vi "Test Semaphore 2.vi"() -> ()   [LabVIEW 2011]
panel:
  out "Iterations":u32
  in  "milliseconds to Hold":u32=500
  in  "milliseconds to wait":u32=500
  out "Wait Time":u32
  out "Hold Time":u32
  out "millisecond timer value 1":u32
  out "Prior Count":i32
  out "millisecond timer value 2":u32
  out "Locked 1":bool
  out "Numeric":i32
  out "Timed Out? 1":bool
  out "error out rel 2":errorcluster
  out "error out acq 2":errorcluster
  in  "Acq":bool
  in  "Release":bool
  in  "stop":bool
  out "Handle":u16
  out "error out create":errorcluster
  in  "Name":string="LabVIEW_System_Semaphore"
  out "error out destroy 1":errorcluster
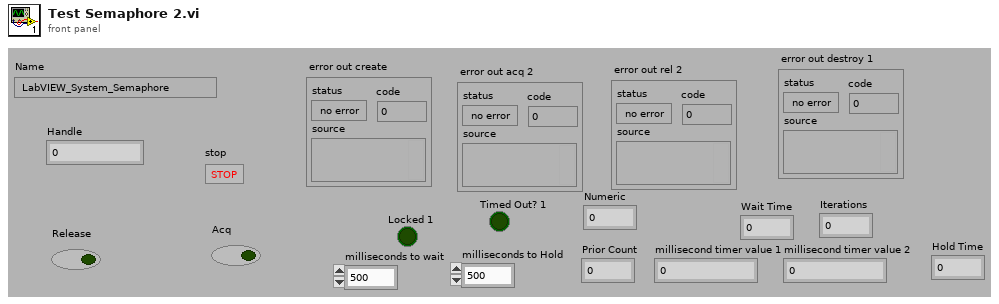
[diagram p1: front panel]
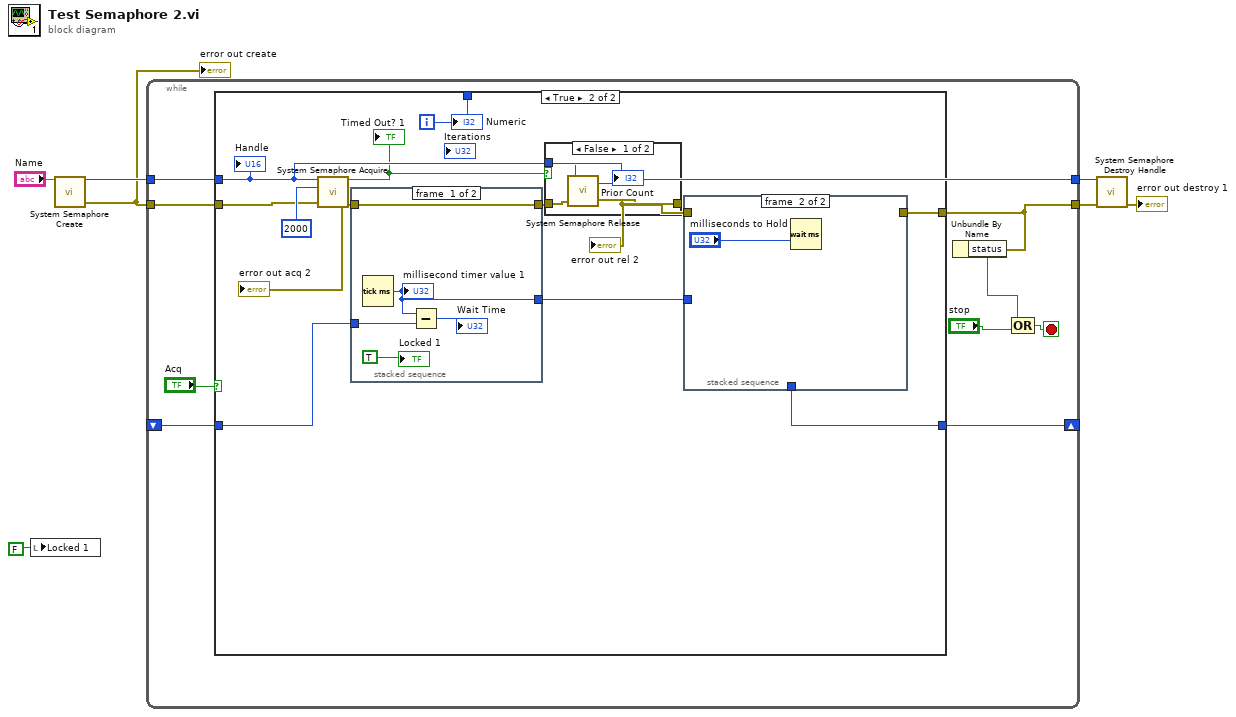
[diagram p0: block diagram]
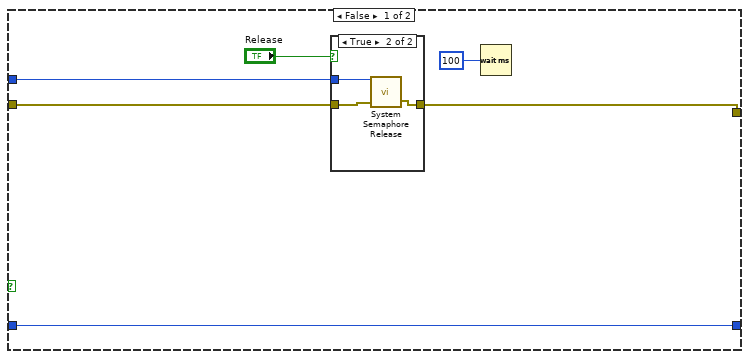
[diagram p2: hidden frame]
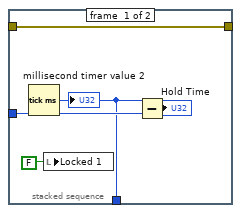
[diagram p5: hidden frame]
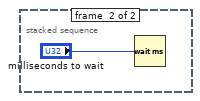
[diagram p6: hidden frame]
diagram:
  n1 = local write "Locked 1"(FALSE) -> ()
  n2 = call "System Semaphore Create.vi"("Name"="Name") -> ("error out"=w2:errorcluster, "Handle"=w7:u16)  [unwired: 4 in]
  "error out create" <- w2
  n3 = while {
    tunnel: w2 -> [w10]
    tunnel: w7 -> [w13]
    tunnel: [w13] -> w6
    tunnel: [w12] -> w5
    shift-right: [w9] -> _
    shift-left: _ -> [w8]
    i -> [w14]
    stop <- w16 stop-if-true
    n4 = case shown="True" "Acq" {
      tunnel: w14 -> [_ w39]
      tunnel: w13 -> [w19 w33]
      tunnel: [w20 w37] -> w12
      tunnel: w10 -> [w21 w32]
      tunnel: [w22 w30] -> w9
      tunnel: w8 -> [w22 w29]
      frame False {
        n5 = case shown="True" "Release" {
          tunnel: w21 -> [w24 w27]
          tunnel: [w24 w26] -> w20
          tunnel: w19 -> [_ w25]
          frame False {
          }
          frame True {
            n6 = call "System Semaphore Release.vi"("error in (no error)"=w27, "SemaphoreHandle"=w25) -> ("error out"=w26:errorcluster)  [unwired: 1 in, 1 out]
          }
        }
        n7 = Wait (ms)(milliseconds to wait=u32 100) -> ()  [unwired: 1 out]
      }
      frame True {
        n8 = call "System Semaphore Acquire.vi"("error in (no error)"=w32, "Timeout (ms)"=u16 2000, "SemaphoreHandle"=w33) -> ("error out"=w36:errorcluster, "Timed Out?"=w28:bool)
        "Timed Out? 1" <- w28
        "error out acq 2" <- w36
        n9 = stacked-sequence {
          tunnel: w36 -> [w55 _]
          tunnel: [w55 _] -> w35
          tunnel: [w52 _] -> w31
          tunnel: w29 -> [w51 _]
          frame #0 {
            n10 = Tick Count (ms)() -> (millisecond timer value=w52:u32)
            "millisecond timer value 1" <- w52
            n11 = Subtract(x=w52, y=w51) -> (x-y=→"Wait Time":u32)
            "Locked 1" <- TRUE
          }
          frame #1 {
            n12 = Wait (ms)(milliseconds to wait="milliseconds to wait") -> ()  [unwired: 1 out]
          }
        }
        n13 = case shown="False" w28 {
          tunnel: w35 -> [w43 w44]
          tunnel: w33 -> [w42 _]
          tunnel: [w41 w44] -> w34
          frame False {
            n14 = call "System Semaphore Release.vi"("error in (no error)"=w43, "SemaphoreHandle"=w42) -> ("error out"=w41:errorcluster, "PreviousCount"=→"Prior Count":i32)  [unwired: 1 in]
          }
          frame True {
          }
        }
        "error out rel 2" <- w34
        n15 = stacked-sequence {
          tunnel: w34 -> [w49 _]
          tunnel: [w49 _] -> w37
          tunnel: w31 -> [w47 _]
          tunnel: [w45 _] -> w30
          frame #0 {
            n16 = Tick Count (ms)() -> (millisecond timer value=w45:u32)
            "millisecond timer value 2" <- w45
            n17 = local write "Locked 1"(FALSE) -> ()
            n18 = Subtract(x=w45, y=w47) -> (x-y=→"Hold Time":u32)
          }
          frame #1 {
            n19 = Wait (ms)(milliseconds to wait="milliseconds to Hold") -> ()  [unwired: 1 out]
          }
        }
        "Handle" <- w33
        "Numeric" <- w39
      }
    }
    n20 = Unbundle By Name(w12) -> ("status"=w15:bool)
    n21 = Compound Arithmetic op=OR(w15, "stop") -> (w16:bool)
  }
  n22 = call "System Semaphore Destroy Handle.vi"("error in (no error)"=w5, "SemaphoreHandle"=w6) -> ("error out"=→"error out destroy 1":errorcluster)  [unwired: 9 in]
